vi "GlobalFan1.vi"() -> ()   [LabVIEW 2024]
panel:
  out "Fan1":bool
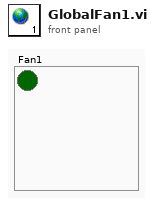
[diagram p1: front panel]
diagram:
